vi "Create Theme.vi"(8 "error in (no error)":errorcluster) -> (0 "error out":errorcluster, 3 "Theme out":refnum<class "Theme.lvclass">)   [LabVIEW 2017, in "Theme.lvlib" / "Theme.lvclass"]
uses:
  Theme.lvclass
  Private Data.ctl
  Theme.Colors/Theme.Colors.lvclass
  Theme.Font/Theme.Font.lvclass
  Theme.lvclass/Theme.ctl
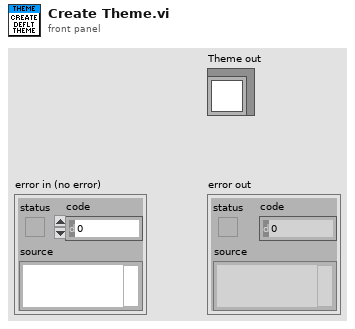
[diagram p1: front panel]
types:
  T1 = typedef "Theme.lvlib/Theme.lvclass/Private Data.ctl" = cluster{"Colors":refnum<class "Theme.Colors.lvclass">, "Font":refnum<class "Theme.Font.lvclass">}
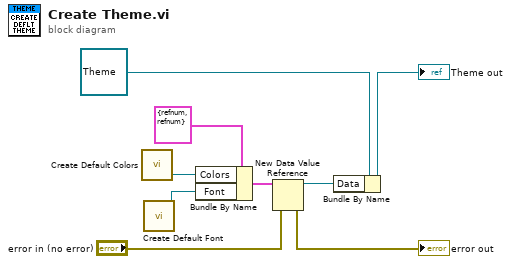
[diagram p0: block diagram]
diagram:
  n1 = call "Create Default Colors.vi"() -> ("Theme.Colors out"=w1:refnum<class "Theme.Colors.lvclass">)  [unwired: 11 in]
  n2 = call "Create Default Font.vi"() -> ("Theme.Font out"=w2:refnum<class "Theme.Font.lvclass">)  [unwired: 11 in]
  n3 = Bundle By Name(cluster=T1 {"Colors"=refnum, "Font"=refnum} ("Private Data"), "Colors"=w1, "Font"=w2) -> (w7:T1)
  n4 = New Data Value Reference(data value=w7, error in="error in (no error)") -> (data value reference=w5:refnum<data-value>, error out=→"error out":errorcluster)
  n5 = Bundle By Name(cluster=refnum<class "Theme.lvclass"> refnum ("Theme in"), "Data"=w5) -> (→"Theme out":refnum<class "Theme.lvclass">)
